vi "LV_2_TDMS.vi"(8 "error in (no error)":errorcluster, 10 "data":T1[](array[typedef]), 11 "file path":path) -> (0 "error out":errorcluster)   [LabVIEW 2016, in "VCL_2_DSC.lvclass"]
uses:
  VCL_2_DSC.lvclass
  typedefs/TSLtoLV-cluster.ctl
  <vilib>/measure/maresamp.llb/Resample Pair of Arrays (single shot).vi
  <vilib>/measure/NI_MAPro.lvlib
panel:
  out "time stamp":timestamp[](array[timestamp])
  out "Array":dbl[](array[numeric])
  out "Waveform Graph":waveform(dbl)[](graph)
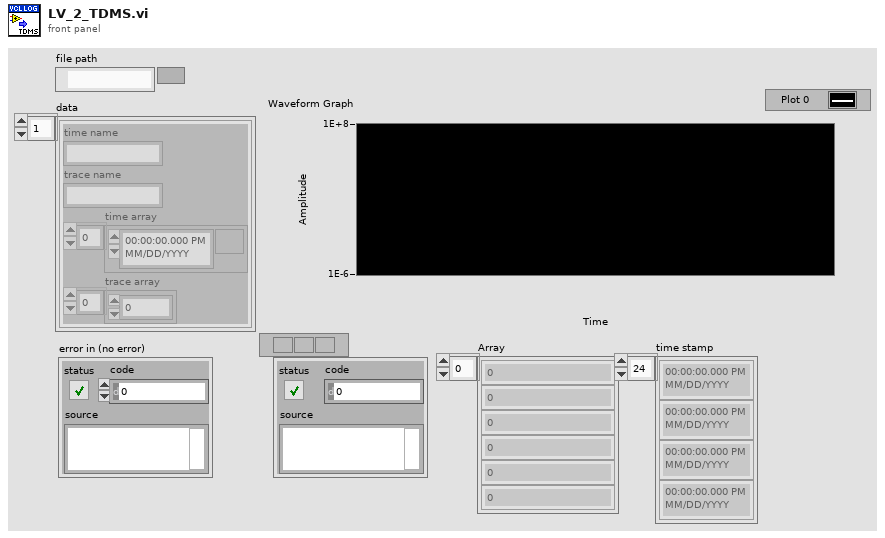
[diagram p1: front panel]
types:
  T1 = typedef "VCL_2_DSC.lvclass/TSLtoLV-cluster.ctl" = cluster{"time name":string, "trace name":string, "time array":timestamp[], "trace array":dbl[]}
  T2 = enum16{"open", "open or create", "create or replace", "create", "open (read-only)"}
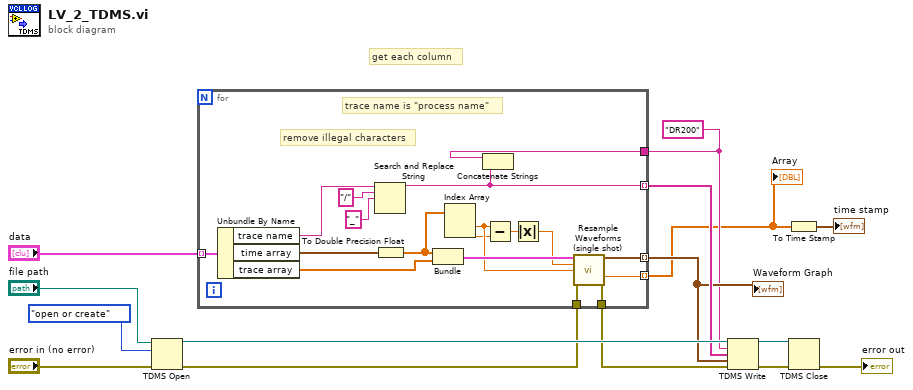
[diagram p0: block diagram]
diagram:
  w3 = "DR200" ("process name")
  # "get each column"
  n1 = TDMS Open(8:"error in (no error)", 10:T2."open or create" ("operation (0:open)"), 11:"file path") -> (0:w5:errorcluster, 3:w10:refnum<k34>)  [unwired: 4 in]
  n2 = for {
    tunnel: "data" -> [w29] mode=indexing
    tunnel: [w28] -> w8 mode=indexing
    tunnel: [w25] -> w6 mode=indexing
    tunnel: w5 -> [w21]
    tunnel: [w20] -> w4
    tunnel: [w19] -> w2 mode=indexing
    tunnel: w3 -> [w18]
    # "trace name is \"process name\""
    # "remove illegal characters"
    n3 = Unbundle By Name(w29) -> ("trace name"=w31:string, "time array"=w30:timestamp[], "trace array"=w26:dbl[])
    n4 = Search and Replace String(input string=w31, search string="/", replace string="_" ("replace string (\"\")")) -> (result string=w28:string)  [unwired: 5 in, 3 out]
    n5 = To Double Precision Float(number=w30) -> (double precision float=w24:dbl[])
    n6 = Bundle(w24, "trace array"=w26) -> (w27:cluster{dbl[], "trace array":dbl[]})  [unwired: 1 in]
    n7 = Index Array(array=w24) -> (element #1=w23:dbl, element #2=w22:dbl)  [unwired: 2 in]
    n8 = Concatenate Strings(w18, w28) -> ()  [unwired: 1 out]
    n9 = Subtract(x=w23, y=w22) -> (x-y=w17:dbl)
    n10 = Absolute Value(x=w17) -> (abs(x)=w16:dbl)
    n11 = call-poly <vilib>:"Resample Waveforms (single shot).vi"("XY-data in"=w27, "dt"=w16, "t0"=w23, "error in (no error)"=w21) -> ("resampled waveform out"=w25:waveform(dbl), "used t0"=w19:dbl, "error out"=w20:errorcluster)  [unwired: 7 in, 2 out]
  }
  "Waveform Graph" <- w6
  "Array" <- w2
  n12 = TDMS Write(0:w10, 5:w3, 7:w8, 9:w6, 11:w4) -> (4:w9:refnum<k34>, 15:w11:errorcluster)  [unwired: 1 in, 2 out]
  n13 = To Time Stamp(1:w2) -> (0:→"time stamp":timestamp[])
  n14 = TDMS Close(8:w11, 11:w9) -> (0:→"error out":errorcluster)  [unwired: 1 out]
